vi "Harmonics.vi"(8 "error in":errorcluster, 9 "complex spectrum":cluster{"f0":dbl, "df":dbl, "spectrum":cdb[]}, 10 "electrical frequency [Hz]":dbl=-1.0, 11 "maximum harmonic":i32=20) -> (0 "error out":errorcluster, 2 "harmonic phase lags":T1, 3 "harmonic levels":cluster{"harmonics":dbl[], "rms levels":dbl[]})   [LabVIEW 2021]
uses:
  <vilib>/Analysis/NI_AALPro.lvlib
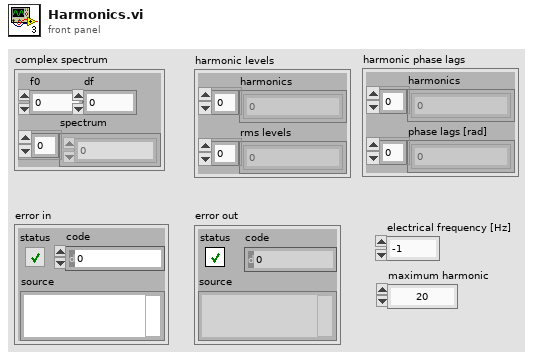
[diagram p1: front panel]
types:
  T1 = cluster{"harmonics":dbl[], "phase lags [rad]":dbl[]}
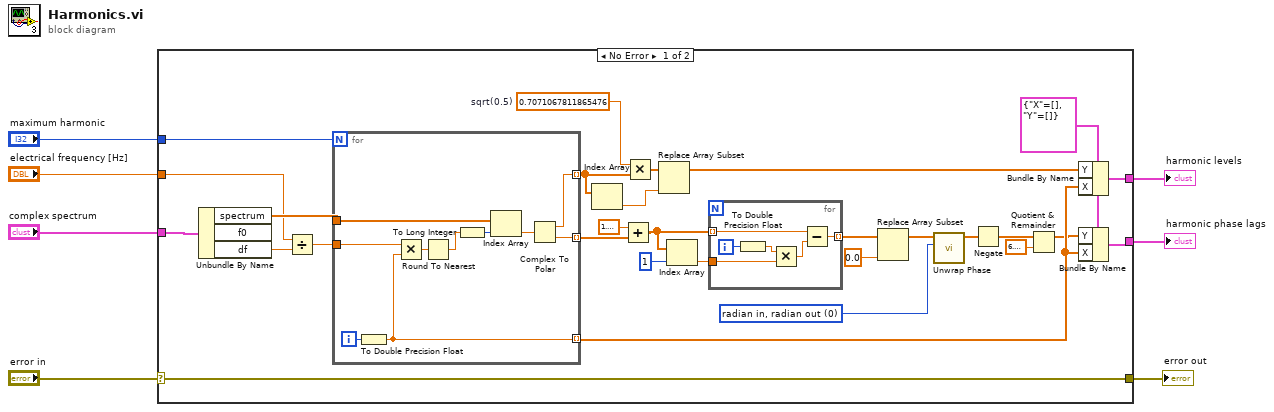
[diagram p0: block diagram]
diagram:
  n1 = case shown="No Error" "error in" {
    selector: "error in" -> [w11 w53]
    tunnel: "maximum harmonic" -> [w8 _]
    tunnel: "electrical frequency [Hz]" -> [w9 _]
    tunnel: [w11 w53] -> w4
    tunnel: [w13 _] -> w3
    tunnel: [w12 _] -> w2
    tunnel: "complex spectrum" -> [w10 _]
    frame No Error {
      w18 = 0 items=["radian in, radian out", "radian in, degree out", "degree in, degree out", "degree in, radian out"] ("phase unit")
      w31 = 0.7071067811865476  # sqrt(0.5)
      w33 = cluster{"X":dbl[], "Y":dbl[]} {"X"=[], "Y"=[]} ("cluster")
      n2 = Unbundle By Name(w10) -> ("spectrum"=w35:cdb[], "df"=w36:dbl)  [unwired: 1 out]
      n3 = Divide(x=w9, y=w36) -> (x/y=w34:dbl)
      n4 = for {
        N: w8 -> [_]
        tunnel: w34 -> [w52]
        tunnel: w35 -> [w50]
        tunnel: [w44] -> w29 mode=indexing
        tunnel: [w46] -> w26 mode=indexing
        tunnel: [w45] -> w30 mode=indexing
        i -> [w51]
        n5 = To Double Precision Float(number=w51) -> (double precision float=w44:dbl)
        n6 = Multiply(x=w52, y=w44) -> (x*y=w49:dbl)
        n7 = Round To Nearest(number=w49) -> (nearest integer value=w43:dbl)
        n8 = To Long Integer(number=w43) -> (32bit integer=w48:i32)
        n9 = Index Array(array=w50, index=w48) -> (element=w47:cdb)
        n10 = Complex To Polar(r * e^(i*theta)=w47) -> (r=w46:dbl, theta=w45:dbl)
      }
      n11 = Index Array(array=w26) -> (element=w25:dbl)  [unwired: 1 in]
      n12 = Add(x=1.5707963267948966, y=w30) -> (x+y=w15:dbl[])
      n13 = Multiply(x=w31, y=w26) -> (x*y=w28:dbl[])
      n14 = Replace Array Subset(array=w28, new element=w25) -> (w27:dbl[])  [unwired: 1 in]
      n15 = Index Array(array=w15, index=1) -> (element=w19:dbl)
      n16 = for {
        tunnel: w15 -> [w42] mode=indexing
        tunnel: w19 -> [w41]
        tunnel: [w39] -> w20 mode=indexing
        i -> [w38]
        n17 = To Double Precision Float(number=w38) -> (double precision float=w37:dbl)
        n18 = Multiply(x=w37, y=w41) -> (x*y=w40:dbl)
        n19 = Subtract(x=w42, y=w40) -> (x-y=w39:dbl)
      }
      n20 = Replace Array Subset(array=w20, new element=0.0 ("new element/subarray")) -> (w21:dbl[])  [unwired: 1 in]
      n21 = call <vilib>:"Unwrap Phase.vi"("phase unit"=w18, "Phase"=w21) -> ("Unwrapped Phase"=w14:dbl[])  [unwired: 8 in, 1 out]
      n22 = Negate(x=w14) -> (-x=w23:dbl[])
      n23 = Quotient & Remainder(x=w23, y=6.283185307179586) -> (x-y*floor(x/y)=w22:dbl[])  [unwired: 1 out]
      n24 = Bundle By Name(cluster=w33, "Y"=w27, "X"=w29) -> (w13:cluster{"X":dbl[], "Y":dbl[]})
      n25 = Bundle By Name(cluster=w33, "Y"=w22, "X"=w29) -> (w12:cluster{"X":dbl[], "Y":dbl[]})
    }
    frame Error {
    }
  }
  "error out" <- w4
  "harmonic levels" <- w3
  "harmonic phase lags" <- w2
